vi "Dequeue.vi"(8 "Error In":errorcluster, 9 "timeout (ms) (Default = -1)":i32=-1) -> (0 "Error Out":errorcluster, 2 "Data":variant, 3 "Command":T1)   [LabVIEW 2023, in "Anti-Spam Tester (AST).lvlib" / "AST MHL Queue.lvclass"]
doc: "Receives a command and feeds it to the module Message Handling Loop (MHL)."
uses:
  AST MHL Queue.lvclass
  Command (enum).ctl
  Queue Reference (library variable).vi
  AST MHL Queue.lvclass/AST MHL Queue.ctl
panel:
  # "Input\nInputs to the VI"
  # "Development\nControls or indicators that are useful for development or testing, but which are not outputs of the VI."
  # "Output\nOutputs of the VI"
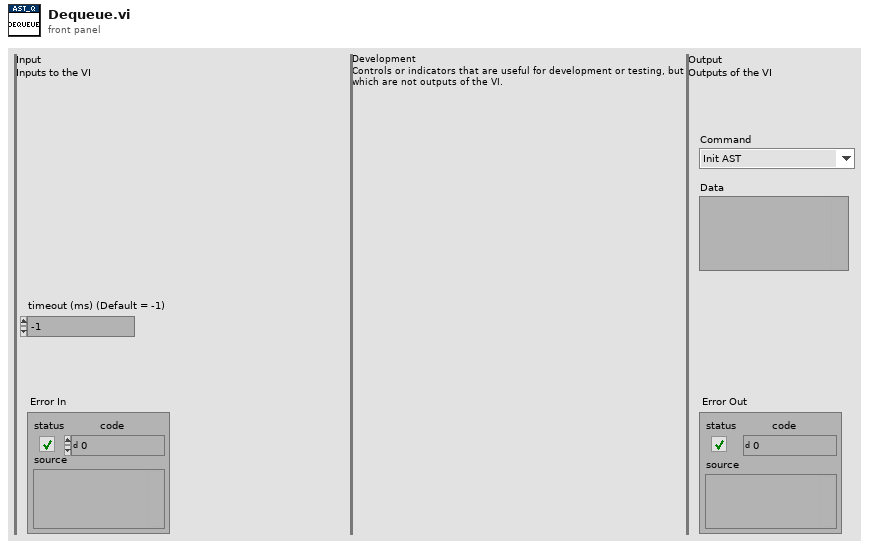
[diagram p1: front panel]
types:
  T1 = typedef "Anti-Spam Tester (AST).lvlib/AST MHL Queue.lvclass/Command (enum).ctl" = enum16{"Init AST", "Close AST", "Config GUI - Init", "Config GUI - Spamming Has Started", "Config GUI - Spamming Has Stopped", "Spam"}
  T2 = typedef "Error Manager.lvlib/Testers.lvlib/Anti-Spam Tester.lvlib/AST MHL Queue.lvlib/Message (cluster).ctl" = cluster{"Command":T3, "Data":variant}
  T3 = typedef "Error Manager.lvlib/Testers.lvlib/Anti-Spam Tester.lvlib/AST MHL Queue.lvlib/Command (enum).ctl" = enum16{"Init AST", "Close AST", "Config GUI - Init", "Config GUI - Spamming Has Started", "Config GUI - Spamming Has Stopped", "Spam"}
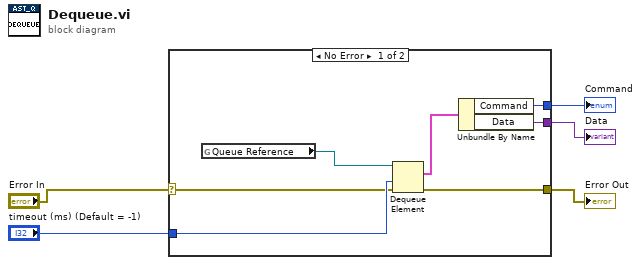
[diagram p0: block diagram]
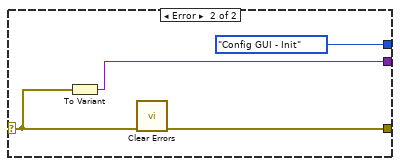
[diagram p2: hidden frame]
diagram:
  n1 = case shown="No Error" "Error In" {
    selector: "Error In" -> [w8 w14]
    tunnel: [w12 w13] -> w5
    tunnel: "timeout (ms) (Default = -1)" -> [w11 _]
    tunnel: [w10 Command_(enum)."Config GUI - Init" ("Command")] -> w3
    tunnel: [w9 w15] -> w2
    frame No Error {
      n2 = global read "Queue Reference (library variable).vi" "Queue Reference"() -> (w6:refnum<queue>)
      n3 = Dequeue Element(queue=w6, timeout in ms (-1)=w11, error in (no error)=w8) -> (element=w7:T2, error out=w12:errorcluster)  [unwired: 2 out]
      n4 = Unbundle By Name(w7) -> ("Command"=w10:T3, "Data"=w9:variant)
    }
    frame Error {
      n5 = To Variant(anything=w14) -> (Variant=w15:variant)
      n6 = call <vilib>:"Clear Errors.vi"("error in (no error)"=w14) -> ("error out"=w13:errorcluster)  [unwired: 5 in, 1 out]
    }
  }
  "Error Out" <- w5
  "Command" <- w3
  "Data" <- w2
